vi "oa_Continuous Convolution.vi"(6 "initial state":dbl[](array[numeric]) format="%.2f", 8 "error in (no error)":errorcluster, 10 "filter coefficients":dbl[](array[numeric]) format="%.2f", 11 "X":dbl[](array[numeric]) format="%.2f") -> (0 "error out":errorcluster, 3 "Y":dbl[](array[numeric]) format="%.2f", 4 "final state":dbl[](array[numeric]) format="%.2f")   [LabVIEW 2017]
uses:
  <vilib>/Analysis/2dsp.llb/1D Convolution (DBL).vi
  <vilib>/Analysis/NI_AALPro.lvlib
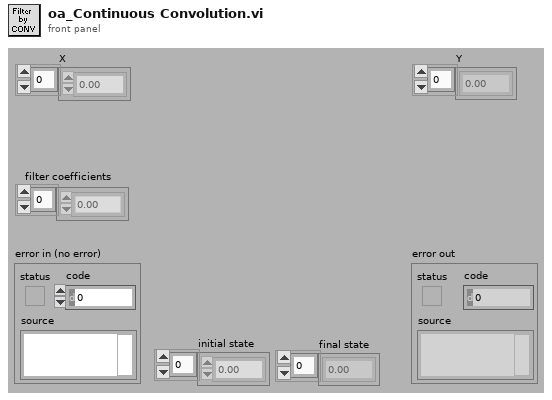
[diagram p1: front panel]
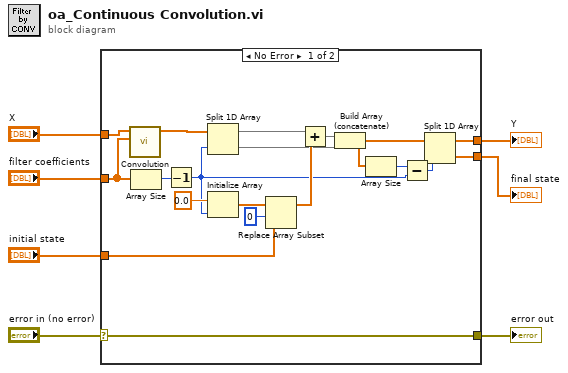
[diagram p0: block diagram]
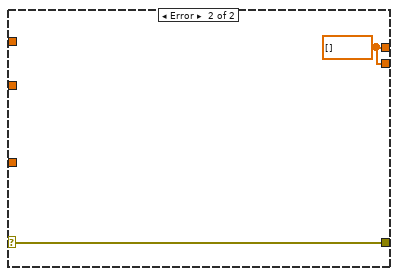
[diagram p2: hidden frame]
diagram:
  n1 = case shown="No Error" "error in (no error)" {
    selector: "error in (no error)" -> [w8 w27]
    tunnel: "X" -> [w26 _]
    tunnel: "filter coefficients" -> [w25 _]
    tunnel: "initial state" -> [w20 _]
    tunnel: [w10 w28] -> w3
    tunnel: [w9 w28] -> w2
    tunnel: [w8 w27] -> w1
    frame No Error {
      n2 = call-poly <vilib>:"Convolution.vi"("Y"=w25, "X"=w26) -> ("X * Y"=w23:dbl[])  [unwired: 8 in, 1 out]
      n3 = Array Size(array=w25) -> (size(s)=w24:i32)
      n4 = Decrement(x=w24) -> (x-1=w13:i32)
      n5 = Split 1D Array(array=w23, index=w13) -> (first subarray=w22:dbl[], second subarray=w15:dbl[])
      n6 = Initialize Array(0.0 ("element"), w13) -> (w19:dbl[])
      n7 = Replace Array Subset(array=w19, new element=w20, index=0) -> (w17:dbl[])
      n8 = Add(x=w22, y=w17) -> (x+y=w16:dbl[])
      n9 = Build Array (concatenate)(w16, w15) -> (w11:dbl[])
      n10 = Array Size(array=w11) -> (size(s)=w14:i32)
      n11 = Subtract(x=w14, y=w13) -> (x-y=w12:i32)
      n12 = Split 1D Array(array=w11, index=w12) -> (first subarray=w10:dbl[], second subarray=w9:dbl[])
    }
    frame Error {
      w28 = dbl[] []
    }
  }
  "Y" <- w3
  "final state" <- w2
  "error out" <- w1
